vi "Robot Global Data.vi"() -> ()   [LabVIEW 2020]
doc: "This global VI can contain as many global variables as you need. Place a control on the panel, give it a good name. To read or write to it from a VI, drag the icon to the diagram of that VI. You can also drag from the project. Click on the node to change which global you access. You shouldn't have multiple locations writing to a global or it will cause a race-condition."
uses:
  <vilib>/Rock Robotics/WPI/Camera/WPI_CameraImageSize.ctl
  <vilib>/Rock Robotics/WPI/DriverStation/WPI_DriverStationRobotMode2.ctl
panel:
  in  "SHOOTER wheel diameter (in)":dbl=6.0 format="%.3g"
  in  "SHOOTER gear ratio":dbl=1.0 format="%.3g"
  in  "NEO ticks/rev":i32=42
  in  "Falcon 500 ticks/rev":i32=2048
  in  "arm angle table":T1
  in  "ARM geometry":T2={"gear ratio"={"value"=3.5714, "descr"="gear transfer from NEO to screw shaft"}, "screw tpi"={"value"=12.0, "descr"="threads per inch"}, "shoulder AG"={"value"=6.875, "descr"="ht of shoulder pin above ground"}, "shoulder to CTR"={"value"=4.0, "descr"="shoulder pin to midline of chassis"}, "shoulder to screw 0"={"value"=11.875, "descr"="horizontal distance shoulder to screw 0"}, "screw shuttle AG"={"value"=12.5, "descr"="screw shuttle pin above ground"}, "screw length"={"value"=12.0, "descr"="total travel length of screw"}, "screw to full front"={"value"=5.0, "descr"="distance from 0 to front limit trigger"}, "screw link"={"value"=11.0, "descr"="pin-pin length of connecting link"}, "lower arm length"={"value"=31.5, "descr"="shoulder pin to top of tube"}, "arm top"={"value"=4.625, "descr"="upper arm left above lower arm"}, "shoulder to pin link Y"={"value"=10.75, "descr"="dist along arm shoulder to link"}, "shoulder to pin link X"={"value"=1.5625, "descr"="dist perp to arm ctr line to pin"}, "hook ht"={"value"=5.875, "descr"="hook ht above top of upper arm"}, "hook clear"={"value"=3.0, "descr"="ht above top of upper bar to clear pipe"}} {"hook clear"."value" format="%.3g"; "hook ht"."value" format="%.3g"; "shoulder to pin link X"."value" format="%.3g"; "shoulder to pin link Y"."value" format="%.3g"; "arm top"."value" format="%.3g"; "lower arm length"."value" format="%.3g"; "screw link"."value" format="%.3g"; "screw to full front"."value" format="%.3g"; "screw length"."value" format="%.3g"; "screw shuttle AG"."value" format="%.3g"; "shoulder to screw 0"."value" format="%.3g"; "shoulder to CTR"."value" format="%.3g"; "shoulder AG"."value" format="%.3g"; "screw tpi"."value" format="%.3g"; "gear ratio"."value" format="%.3g"}
  in  "Robot Mode":T3
  in  "image size":T4=enum."320x240"
  in  "Enable Vision":bool
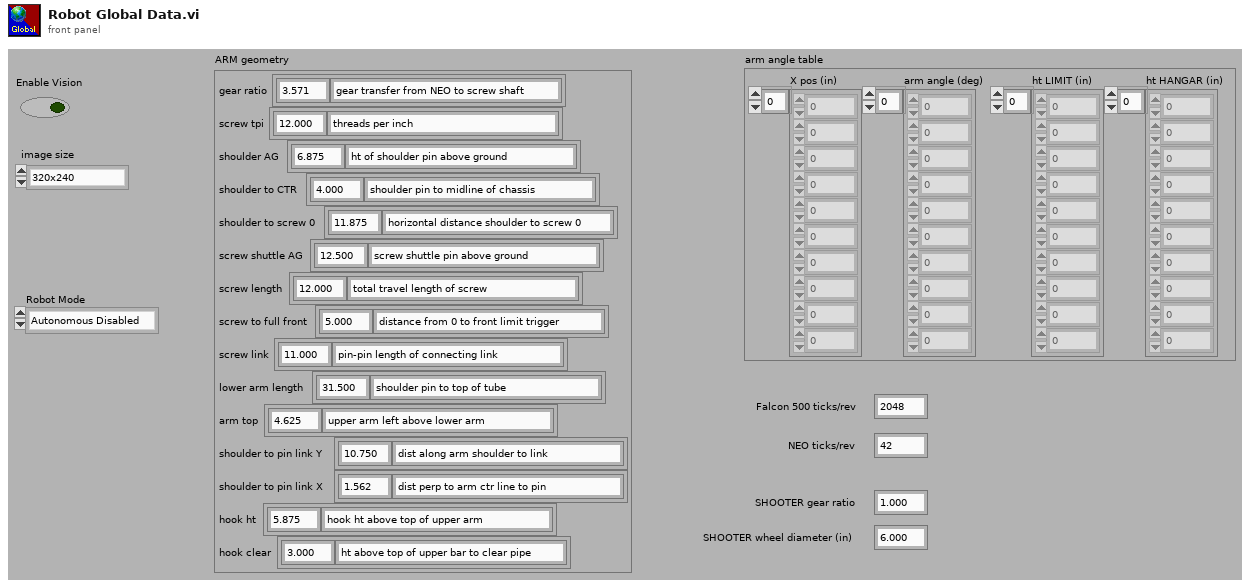
[diagram p1: front panel]
types:
  T1 = cluster{"X pos (in)":dbl[], "arm angle (deg)":dbl[], "ht LIMIT (in)":dbl[], "ht HANGAR (in)":dbl[]}
  T2 = cluster{"gear ratio":cluster{"value":dbl, "descr":string}, "screw tpi":cluster{"value":dbl, "descr":string}, "shoulder AG":cluster{"value":dbl, "descr":string}, "shoulder to CTR":cluster{"value":dbl, "descr":string}, "shoulder to screw 0":cluster{"value":dbl, "descr":string}, "screw shuttle AG":cluster{"value":dbl, "descr":string}, "screw length":cluster{"value":dbl, "descr":string}, "screw to full front":cluster{"value":dbl, "descr":string}, "screw link":cluster{"value":dbl, "descr":string}, "lower arm length":cluster{"value":dbl, "descr":string}, "arm top":cluster{"value":dbl, "descr":string}, "shoulder to pin link Y":cluster{"value":dbl, "descr":string}, "shoulder to pin link X":cluster{"value":dbl, "descr":string}, "hook ht":cluster{"value":dbl, "descr":string}, "hook clear":cluster{"value":dbl, "descr":string}}
  T3 = typedef "WPI_DriverStationRobotMode2.ctl" = enum16{"Autonomous Disabled", "Autonomous Enabled", "Teleop Disabled", "Teleop Enabled", "Disconnected", "Finish", "Test Disabled", "Test Enabled", "Emergency Stopped"}
  T4 = typedef "WPI_CameraImageSize.ctl" = enum16{"640x480", "320x240", "160x120", "Custom"}
diagram:
